vi "UDP Data Engine.vi"(7 "WaveformChart Ref":refnum<vi>, 8 "error in (no error)":errorcluster, 10 "UDP Engine Queue":refnum<queue>, 11 "WorkspaceManager":T1) -> (0 "error out":errorcluster, 1 "Exit":bool, 2 "Update?":bool, 3 "Waveform":waveform(dbl)[](array[waveform]))   [LabVIEW 2019, in "Control Workspace Shared.lvlib"]
uses:
  Types/UDP Streaming Command Cluster.ctl
  Types/UDP Streaming State.ctl
  <vilib>/NI VeriStand/Execution/Workspace/WorkspaceAPI.ctl
  NationalInstruments.VeriStand.ClientAPI
  <vilib>/NI VeriStand/Execution/Workspace/UDPChannelStreamSession.ctl
  <vilib>/NI VeriStand/Execution/Workspace/UDP Stream Packet.ctl
  <vilib>/Utility/tcp.llb/UDP Multicast Read-Only Open.vi
  Control Workspace Shared.lvlib
  <vilib>/NI VeriStand/Execution/Workspace/NI_VS Workspace ExecutionAPI.lvlib
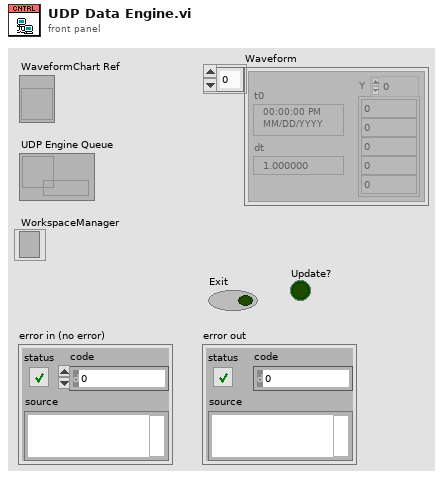
[diagram p1: front panel]
types:
  T1 = typedef "NI_VS Workspace ExecutionAPI.lvlib/WorkspaceAPI.ctl" = refnum<k24>
  T2 = typedef "Control Workspace Shared.lvlib/UDP Streaming State.ctl" = enum8{"Idle", "Start Acq", "Run", "Stop Acq", "Exit"}
  T3 = typedef "NI_VS Workspace ExecutionAPI.lvlib/UDPChannelStreamSession.ctl" = refnum<k24>
  T4 = cluster{"Initialized Waveform":waveform(dbl)[], "VS UDP Session":T3, "Channel IDs":i32[], "Packet IDs":i32[], "Max Packet Size":i32, "UDP Ref":refnum<k16>}
  T5 = typedef "Control Workspace Shared.lvlib/UDP Streaming Command Cluster.ctl" = cluster{"Action":T2, "Channels":string[]}
  T6 = typedef "NI_VS Workspace ExecutionAPI.lvlib/UDP Stream Packet.ctl" = cluster{"ID":i32, "t0":dbl, "dt":dbl, "Channel IDs":i32[], "Channel Data":dbl[][], "Sample Offset":u64}
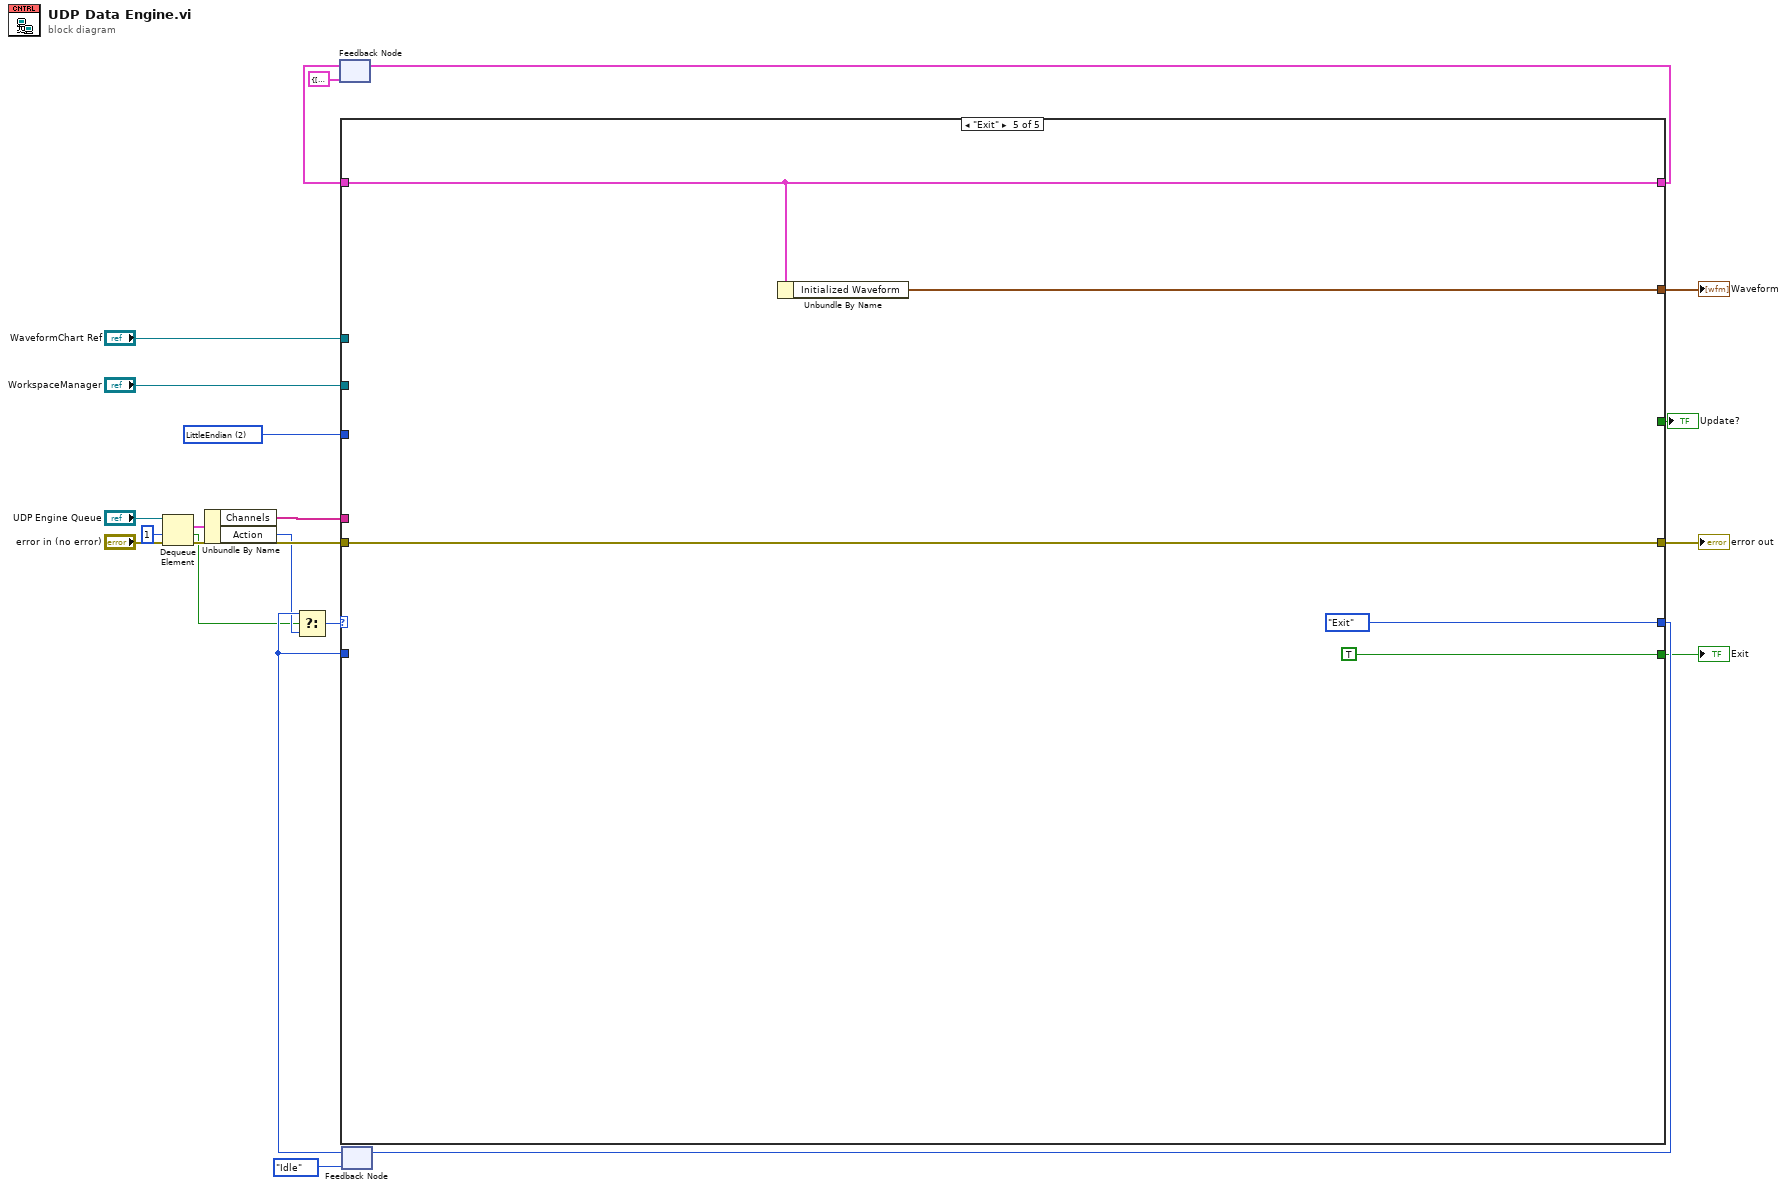
[diagram p0: block diagram]
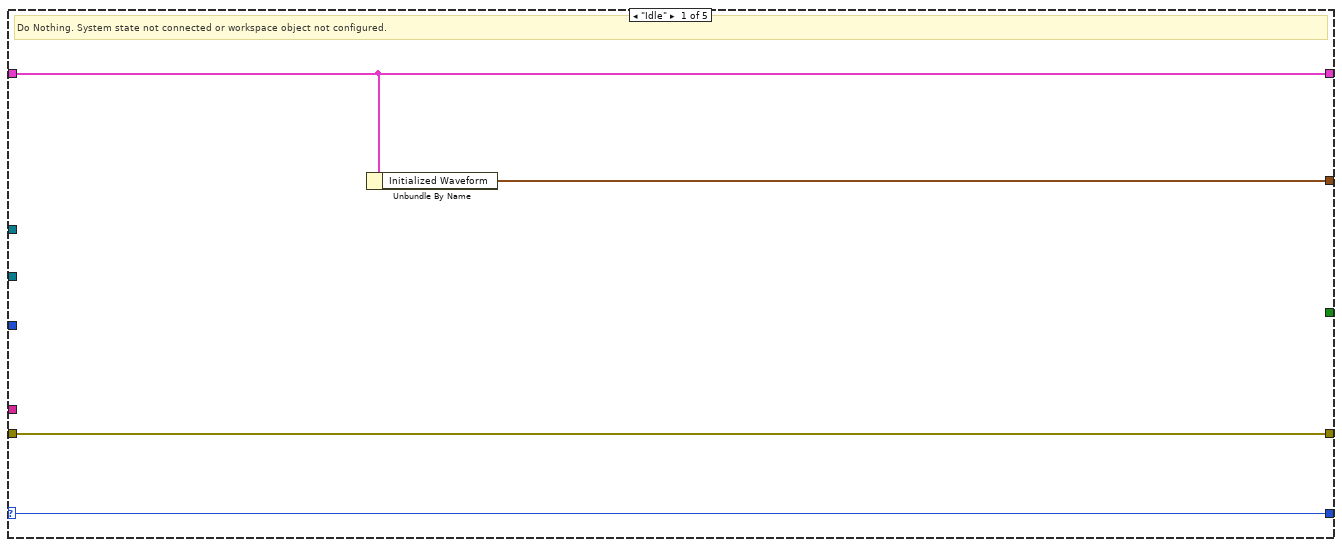
[diagram p2: hidden frame]
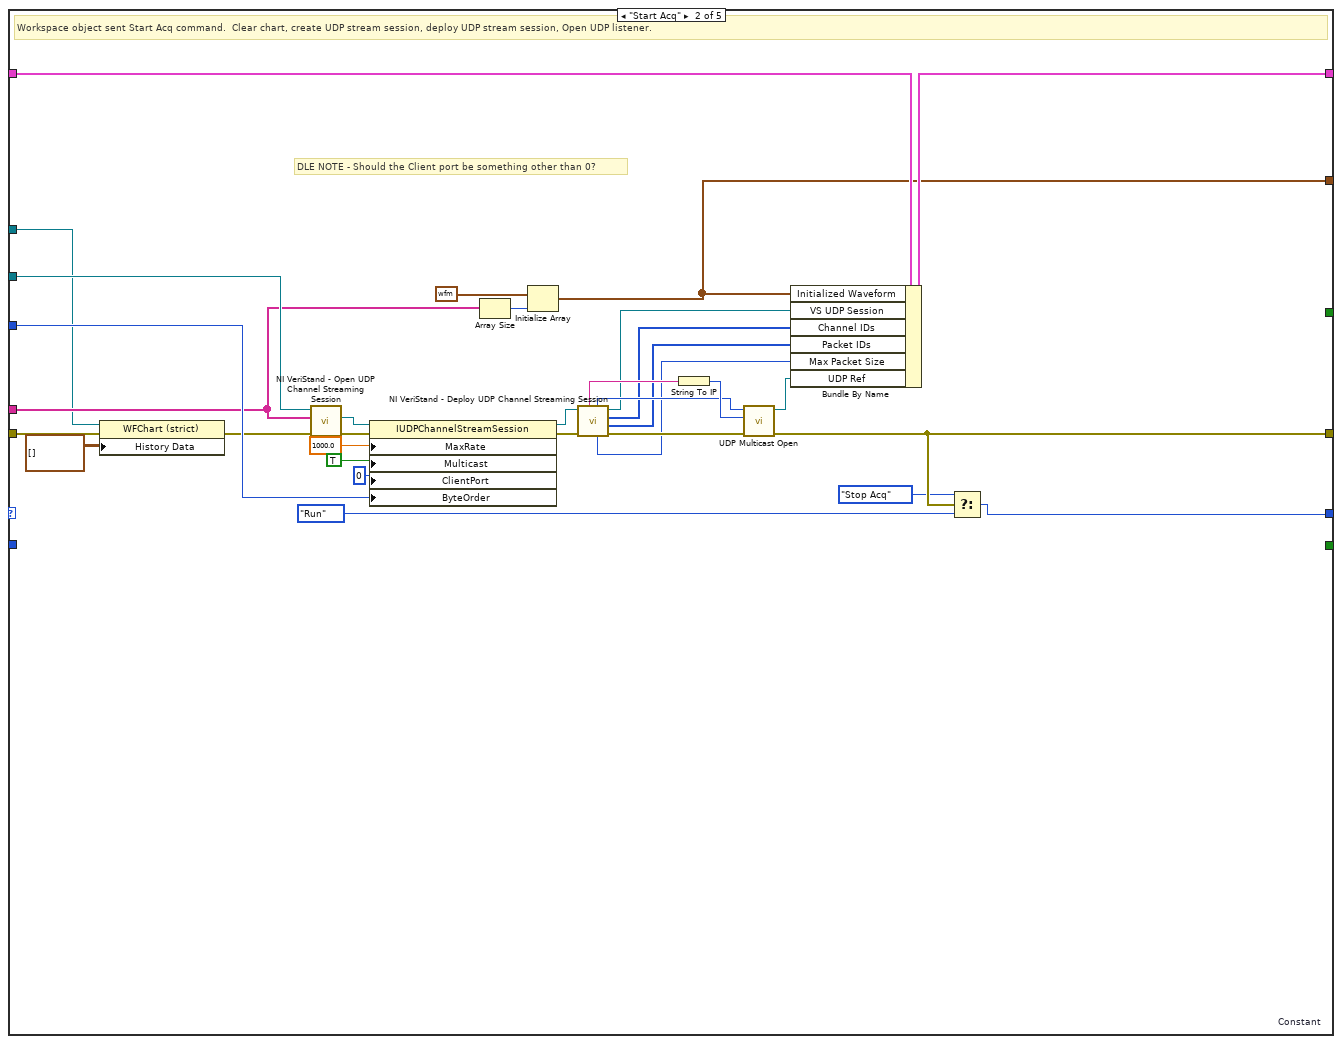
[diagram p3: hidden frame]
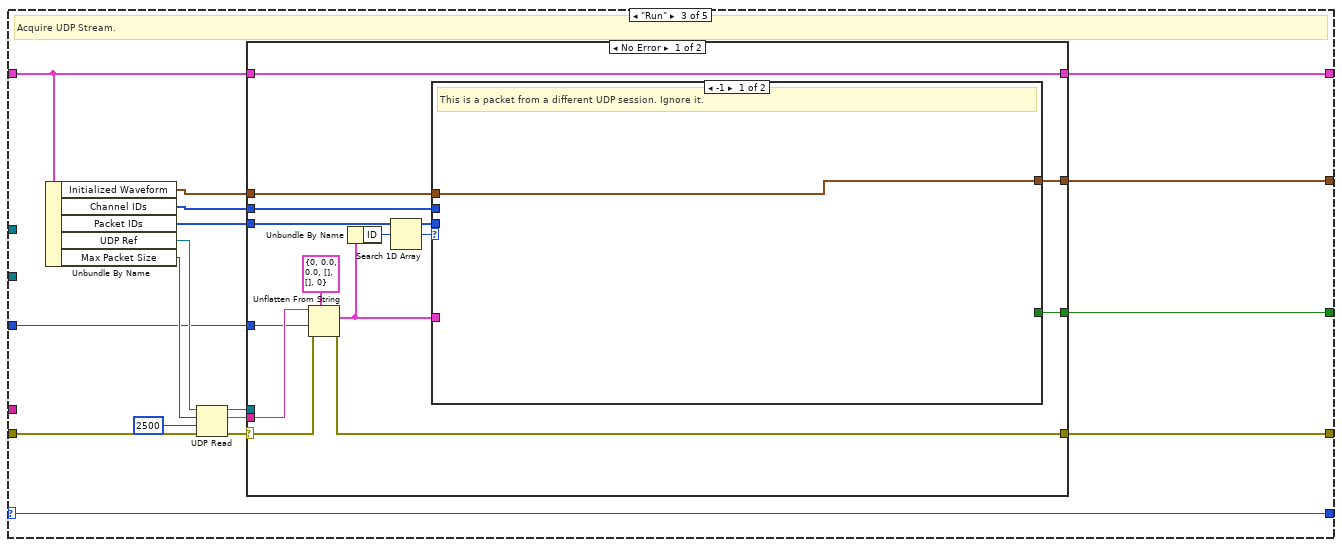
[diagram p4: hidden frame]
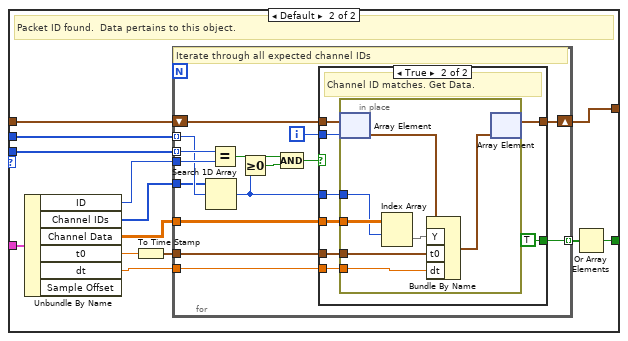
[diagram p5: hidden frame]
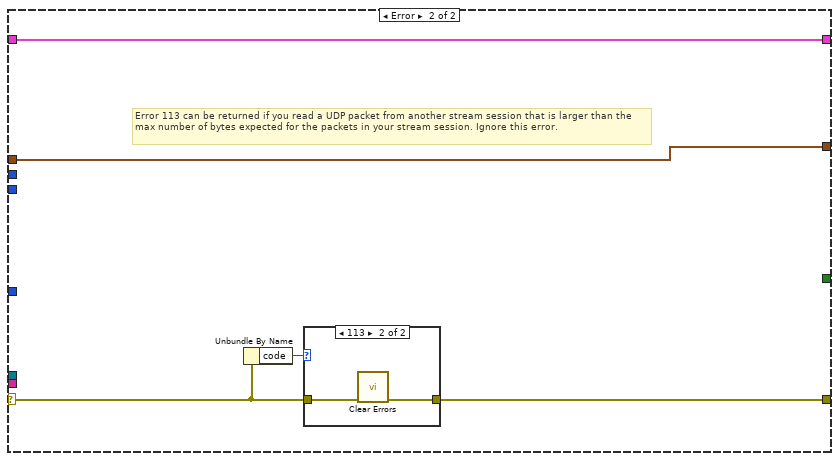
[diagram p7: hidden frame]
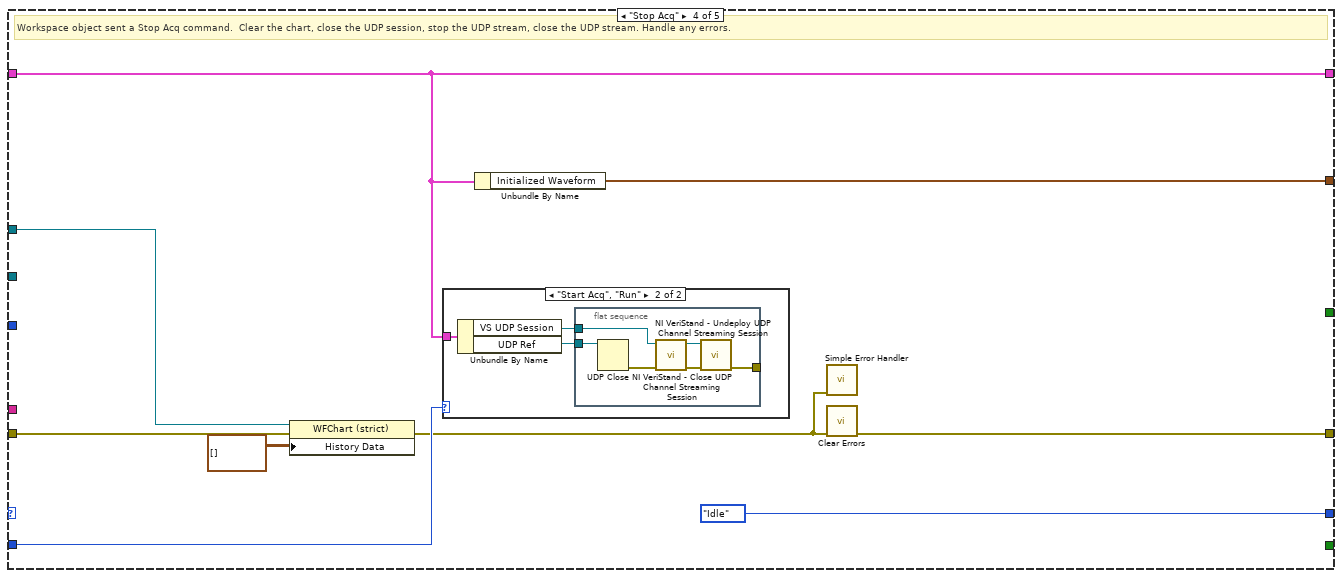
[diagram p9: hidden frame]
diagram:
  w15 = 2 items=["BigEndian", "NativeHostOrder", "LittleEndian"] ("Byte Order")
  n1 = Dequeue Element(queue="UDP Engine Queue", timeout in ms (-1)=1, error in (no error)="error in (no error)") -> (element=w5:T5, timed out?=w7:bool, error out=w11:errorcluster)  [unwired: 1 out]
  n2 = Unbundle By Name(w5) -> ("Channels"=w14:string[], "Action"=w8:T2)
  n3 = feedback #1(T4 {"Initialized Waveform"=[], "VS UDP Session"=refnum, "Channel IDs"=[], "Packet IDs"=[], "Max Packet Size"=0, "UDP Ref"=refnum}) -> (w17:T4)
  n4 = feedback #2(UDP_Streaming_State."Idle" ("Action")) -> (w21:T2)
  n5 = Select(t=w21, s=w7, f=w8) -> (s? t:f=w9:T2)
  n6 = case shown="\"Exit\"" w9 {
    selector: w9 -> [w25 _ w64 _ _]
    tunnel: "WorkspaceManager" -> [_ w46 _ _ _]
    tunnel: w17 -> [w24 w45 w65 w144 w162]
    tunnel: w15 -> [_ w39 w61 _ _]
    tunnel: [w24 w38 w66 w144 w162] -> w16
    tunnel: [w25 w34 w64 UDP_Streaming_State."Idle" ("Action") UDP_Streaming_State."Exit" ("Action")] -> w19
    tunnel: [_ _ _ _ TRUE] -> w10
    tunnel: w11 -> [w26 w28 w63 w146 w163]
    tunnel: [w26 w37 w62 w150 w163] -> w12
    tunnel: w14 -> [_ w32 _ _ _]
    tunnel: w21 -> [_ _ _ w149 _]
    tunnel: [w23 w30 w60 w143 w161] -> w22
    tunnel: "WaveformChart Ref" -> [_ w29 _ w148 _]
    tunnel: [_ _ w59 _ _] -> w1
    frame "Idle" {
      # "Do Nothing. System state not connected or workspace object not configured."
      n7 = Unbundle By Name(w24) -> ("Initialized Waveform"=w23:waveform(dbl)[])
    }
    frame "Start Acq" {
      w52 = waveform(dbl) {"t0"=timestamp(0 s since 1904-01-01), "dt"=1.0, "Y"=[]}  # Constant
      # "DLE NOTE - Should the Client port be something other than 0?"
      # "Workspace object sent Start Acq command.  Clear chart, create UDP stream session, deploy UDP stream session, Open UDP listener."
      n8 = property on="Property Node" class="WFChart (strict)"(reference=w29, error in=w28, "History Data"=waveform(dbl)[][] []) -> (error out=w27:errorcluster)  [unwired: 1 out]
      n9 = call <vilib>:"NI VeriStand - Open UDP Channel Streaming Session.vi"("error in (no error)"=w27, "Channels"=w32, "WorkspaceManager in"=w46) -> ("error out"=w56:errorcluster, "UDPChannelStreamSession out"=w53:T3)  [unwired: 6 in, 1 out]
      n10 = property class="IUDPChannelStreamSession"(reference=w53, error in=w56, "MaxRate"=1000.0, "Multicast"=TRUE, "ClientPort"=u16 0, "ByteOrder"=w39) -> (reference out=w55:T3, error out=w54:errorcluster)
      n11 = Array Size(array=w32) -> (size(s)=w51:i32)
      n12 = Initialize Array(w52, w51) -> (w30:waveform(dbl)[])
      n13 = call <vilib>:"NI VeriStand - Deploy UDP Channel Streaming Session.vi"("error in (no error)"=w54, "UDPChannelStreamSession in"=w55) -> ("error out"=w48:errorcluster, "Packet IDs"=w42:i32[], "Channel IDs"=w43:i32[], "UDPChannelStreamSession out"=w44:T3, "Max Packet Size"=w41:i32, "Port"=w49:u16, "UDP Multicast Address"=w47:string)  [unwired: 3 in]
      n14 = String To IP(1:w47) -> (0:w50:u32)
      n15 = call-poly <vilib>:"UDP Multicast Open.vi"("error in (no error)"=w48, "multicast addr"=w50, "port"=w49) -> ("error out"=w37:errorcluster, "connection ID"=w40:refnum<k16>)  [unwired: 6 in, 1 out]
      n16 = Bundle By Name(cluster=w45, "Initialized Waveform"=w30, "VS UDP Session"=w44, "Channel IDs"=w43, "Packet IDs"=w42, "Max Packet Size"=w41, "UDP Ref"=w40) -> (w38:T4)
      n17 = Select(t=UDP_Streaming_State."Stop Acq", s=w37, f=UDP_Streaming_State."Run" ("Action")) -> (s? t:f=w34:T2)
    }
    frame "Run" {
      # "Acquire UDP Stream."
      n18 = Unbundle By Name(w65) -> ("Initialized Waveform"=w71:waveform(dbl)[], "Channel IDs"=w70:i32[], "Packet IDs"=w69:i32[], "UDP Ref"=w68:refnum<k16>, "Max Packet Size"=w67:i32)
      n19 = UDP Read(connection ID=w68, max size (548)=w67, timeout ms (25000)=2500, 8:w63) -> (data out=w73:string, error out=w74:errorcluster, 3:w75:refnum<k16>)  [unwired: 2 out]
      n20 = case shown="No Error" w74 {
        selector: w74 -> [w88 w136]
        tunnel: w69 -> [w83 _]
        tunnel: w73 -> [w86 _]
        tunnel: w70 -> [w85 _]
        tunnel: w71 -> [w84 w137]
        tunnel: [w89 w138] -> w62
        tunnel: w75 -> [_ _]
        tunnel: w61 -> [w79 _]
        tunnel: [w78 w139] -> w66
        tunnel: w65 -> [w78 w139]
        tunnel: [w77 w137] -> w60
        tunnel: [w76 _] -> w59
        frame No Error {
          n21 = Unflatten From String(type=T6 {"ID"=0, "t0"=0.0, "dt"=0.0, "Channel IDs"=[], "Channel Data"=[], "Sample Offset"=0} ("UDP Data Packet"), binary string=w86, byte order (0:big-endian, network order)=w79, error in (no error)=w88) -> (value=w80:T6, error out=w89:errorcluster)  [unwired: 1 in, 1 out]
          n22 = Unbundle By Name(w80) -> ("ID"=w81:i32)
          n23 = Search 1D Array(1D array=w83, element=w81) -> (index of element=w82:i32)  [unwired: 1 in]
          n24 = case shown="-1" w82 {
            tunnel: w85 -> [_ w103]
            tunnel: w84 -> [w90 w102]
            tunnel: w83 -> [_ w100]
            tunnel: w80 -> [_ w99]
            tunnel: [w90 w93] -> w77
            tunnel: [_ w91] -> w76
            frame -1 {
              # "This is a packet from a different UDP session. Ignore it."
            }
            frame Default {
              # "Packet ID found.  Data pertains to this object."
              n25 = Unbundle By Name(w99) -> ("ID"=w98:i32, "Channel IDs"=w97:i32[], "Channel Data"=w96:dbl[][], "t0"=w95:dbl, "dt"=w94:dbl)  [unwired: 1 out]
              n26 = To Time Stamp(1:w95) -> (0:w101:timestamp)
              n27 = for {
                tunnel: w103 -> [w116] mode=indexing
                tunnel: w100 -> [w118] mode=indexing
                tunnel: w98 -> [w117]
                tunnel: w96 -> [w110]
                tunnel: w97 -> [w109]
                shift-right: [w105] -> w93
                shift-left: w102 -> [w108]
                tunnel: w101 -> [w107]
                tunnel: w94 -> [w106]
                tunnel: [w104] -> w92 mode=indexing
                i -> [w111]
                # "Iterate through all expected channel IDs"
                n28 = Search 1D Array(1D array=w109, element=w116) -> (index of element=w112:i32)  [unwired: 1 in]
                n29 = Equal?(x=w118, y=w117) -> (x = y?=w115:bool)
                n30 = Greater Or Equal To 0?(x=w112) -> (x >= 0?=w114:bool)
                n31 = Compound Arithmetic op=AND(w115, w114) -> (w113:bool)
                n32 = case shown="True" w113 {
                  tunnel: w112 -> [_ w125]
                  tunnel: w111 -> [_ w121]
                  tunnel: w110 -> [_ w126]
                  tunnel: w108 -> [w119 w127]
                  tunnel: w107 -> [_ w124]
                  tunnel: w106 -> [_ w123]
                  tunnel: [w119 w122] -> w105
                  tunnel: [_ TRUE] -> w104
                  frame False {
                    # "This channel is not in this UDP Data Packet."
                  }
                  frame True {
                    # "Channel ID matches. Get Data."
                    n33 = in-place {
                      in-place-border: w126 -> [w133]
                      in-place-border: w125 -> [w132]
                      in-place-border: w124 -> [w130]
                      in-place-border: w123 -> [w129]
                      n34 = in-place-array #3(w127, w121) -> (w134:waveform(dbl))
                      n35 = Index Array(array=w133, index (row)=w132) -> (element=w131:dbl[])  [unwired: 1 in]
                      n36 = Bundle By Name(cluster=w134, "Y"=w131, "t0"=w130, "dt"=w129) -> (w128:waveform(dbl))
                      n37 = in-place-array #3(w128) -> (w122:waveform(dbl)[])  [unwired: 1 out]
                    }
                  }
                }
              }
              n38 = Or Array Elements(Boolean array=w92) -> (logical OR=w91:bool)
            }
          }
        }
        frame Error {
          # "Error 113 can be returned if you read a UDP packet from another stream session that is larger than the max number of bytes expected for the packets in your stream session. Ignore this error."
          n39 = Unbundle By Name(w136) -> ("code"=w135:i32)
          n40 = case shown="113" w135 {
            tunnel: [w140 w142] -> w138
            tunnel: w136 -> [w140 w141]
            frame Default {
            }
            frame 113 {
              n41 = call <vilib>:"Clear Errors.vi"("error in (no error)"=w141) -> ("error out"=w142:errorcluster)  [unwired: 5 in, 1 out]
            }
          }
        }
      }
    }
    frame "Stop Acq" {
      # "Workspace object sent a Stop Acq command.  Clear the chart, close the UDP session, stop the UDP stream, close the UDP stream. Handle any errors."
      n42 = property on="Property Node" class="WFChart (strict)"(reference=w148, error in=w146, "History Data"=waveform(dbl)[][] []) -> (error out=w145:errorcluster)  [unwired: 1 out]
      n43 = case shown="\"Start Acq\", \"Run\"" w149 {
        tunnel: w144 -> [_ w152]
        frame Default {
        }
        frame "Start Acq", "Run" {
          n44 = Unbundle By Name(w152) -> ("VS UDP Session"=w153:T3, "UDP Ref"=w154:refnum<k16>)
          n45 = flat-sequence {
            tunnel: w154 -> [w157]
            tunnel: w153 -> [w156]
            tunnel: [w155] -> _
            frame #0 {
              n46 = UDP Close(connection ID=w157) -> (error out=w160:errorcluster)  [unwired: 1 in, 1 out]
              n47 = call <vilib>:"NI VeriStand - Undeploy UDP Channel Streaming Session.vi"("error in (no error)"=w160, "UDPChannelStreamSession in"=w156) -> ("error out"=w158:errorcluster, "UDPChannelStreamSession out"=w159:T3)  [unwired: 8 in]
              n48 = call <vilib>:"NI VeriStand - Close UDP Channel Streaming Session.vi"("error in (no error)"=w158, "UDPChannelStreamSession in"=w159) -> ("error out"=w155:errorcluster)  [unwired: 9 in]
            }
          }
        }
      }
      n49 = Unbundle By Name(w144) -> ("Initialized Waveform"=w143:waveform(dbl)[])
      n50 = call <vilib>:"Simple Error Handler.vi"("error in (no error)"=w145) -> ()  [unwired: 4 in, 5 out]
      n51 = call <vilib>:"Clear Errors.vi"("error in (no error)"=w145) -> ("error out"=w150:errorcluster)  [unwired: 5 in, 1 out]
    }
    frame "Exit" {
      n52 = Unbundle By Name(w162) -> ("Initialized Waveform"=w161:waveform(dbl)[])
    }
  }
  "Waveform" <- w22
  "error out" <- w12
  "Exit" <- w10
  "Update?" <- w1
  n53 = feedback-in #1(w16) -> ()
  n54 = feedback-in #2(w19) -> ()
